vi "Get 项标识符.vi"(11 "LNK in":refnum<class "Menu.lvclass">) -> (2 "项标识符":string, 3 "LNK out":refnum<class "Menu.lvclass">)   [LabVIEW 2016, in "Menu.lvclass"]
uses:
  Menu.lvclass
  Menu.lvclass/Menu.ctl
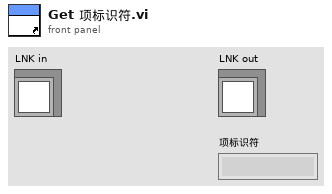
[diagram p1: front panel]
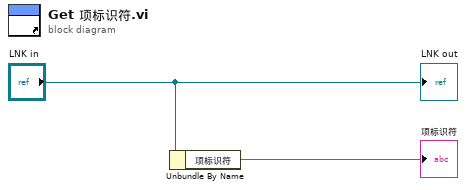
[diagram p0: block diagram]
diagram:
  n1 = Unbundle By Name("LNK in") -> ("项标识符"=→"项标识符":string)
  "LNK out" <- "LNK in"
